vi "Configure Arbitrary Waveform.vi"(0 "RedPitaya connection in":refnum<k5>, 2 "Data":dbl[](array[numeric])=[0.0] min=-1.0 max=1.0, 5 "error in":errorcluster, 8 "Channel #":u16(ring)=1 items=["Channel 1"=1, "Channel 2"=2], 12 "timeout ms (2000)":i32=2000) -> (14 "RedPitaya connection out":refnum<k5>, 19 "error out":errorcluster)   [LabVIEW 2021, in "RedPitaya.lvlib"]
doc: "Send waveform data to Red Pitaya and configures the arbitrary waveform generator."
uses:
  RedPitaya.lvlib
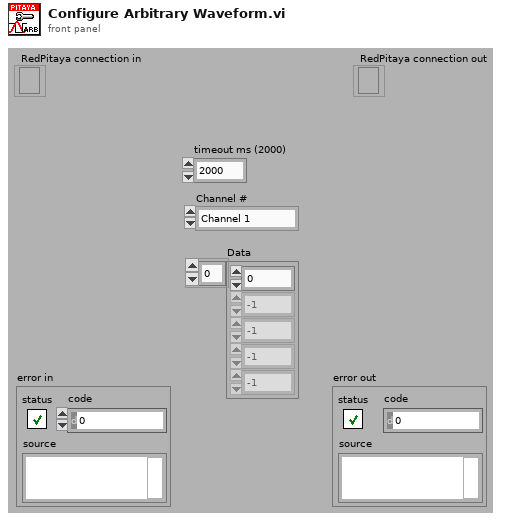
[diagram p1: front panel]
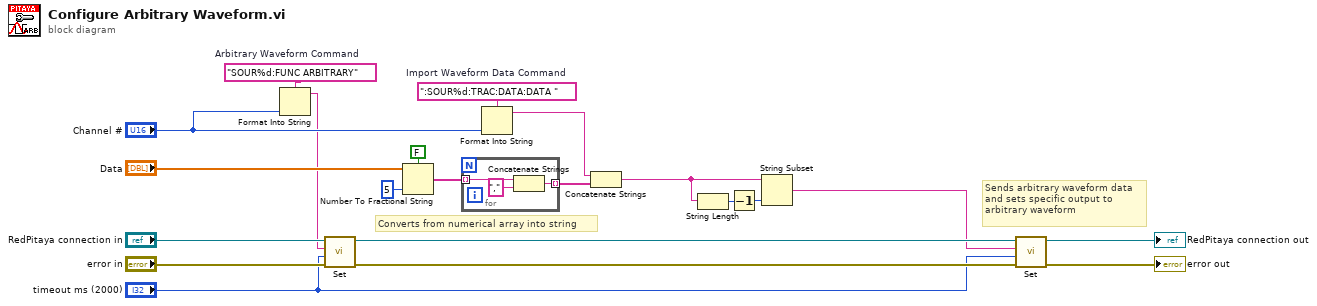
[diagram p0: block diagram]
diagram:
  w14 = "SOUR%d:FUNC ARBITRARY"  # Arbitrary Waveform Command
  w21 = ":SOUR%d:TRAC:DATA:DATA "  # Import Waveform Data Command
  # "Sends arbitrary waveform data\nand sets specific output to \narbitrary waveform"
  # "Converts from numerical array into string"
  n1 = Format Into String(format string=w14, "Channel #") -> (resulting string=w6:string)  [unwired: 2 in, 1 out]
  n2 = call "Set.vi"("error in"="error in", "timeout ms (2000)"="timeout ms (2000)", "SCPI Message"=w6, "RedPitaya connection in"="RedPitaya connection in") -> ("error out"=w8:errorcluster, "RedPitaya connection out"=w10:refnum<k5>)  [unwired: 5 in, 1 out]
  n3 = Number To Fractional String(use system decimal point (T)=FALSE, number="Data", precision (6)=i16 5) -> (F-format string=w16:string[])  [unwired: 1 in]
  n4 = for {
    tunnel: w16 -> [w24] mode=indexing
    tunnel: [w22] -> w18 mode=indexing
    n5 = Concatenate Strings(w24, "," ("string")) -> (w22:string)
  }
  n6 = Format Into String(format string=w21, "Channel #") -> (resulting string=w17:string)  [unwired: 2 in, 1 out]
  n7 = Concatenate Strings(w17, w18) -> (w2:string)
  n8 = String Length(string=w2) -> (length=w4:i32)
  n9 = Decrement(x=w4) -> (x-1=w3:i32)
  n10 = String Subset(string=w2, length (rest)=w3) -> (substring=w1:string)  [unwired: 1 in]
  n11 = call "Set.vi"("error in"=w8, "timeout ms (2000)"="timeout ms (2000)", "SCPI Message"=w1, "RedPitaya connection in"=w10) -> ("error out"=→"error out":errorcluster, "RedPitaya connection out"=→"RedPitaya connection out":refnum<k5>)  [unwired: 5 in, 1 out]
